vi "WireTunnel__slk_mt.vi"(8 "error in (no error)":errorcluster, 10 "vi name":string, 11 "application reference":refnum<vi>) -> (0 "error out":errorcluster)   [LabVIEW 2013, in "Lazyboots Menu Tool.lvlib"]
doc: "This VI is the core of <b>Wire Tunnel</b> function, and will be called by corresponding menu launcher."
uses:
  Library/Lazyboots Menu Tool.lvlib
  Private/WireTunnel/TypeDef_WireTunnelState__slk_mt.ctl
panel:
  # "WireTunnel__slk_mt.vi\nThis VI is the core of <b>Wire Tunnel</b> function, and will be called by corresponding menu launcher.\n\nNOTICE -- YOU MUST LEAVE THIS NOTICE IN PLACE.\n\nCopyright (c) 2011, LIANG LIU Shawn.Liu.cn@gmail.com\nAll rights reserved.\n\nRedistribution and use in source and binary forms, with or without modification, are permitted provided that the following conditions are met:\n-Redistributions of source code must retain the above copyright notice, this list of conditions and the following disclaimer.\n-Redistributions in binary form must reproduce the above copyright notice, this list of conditions and the following disclaimer in the documentation and/or other materials provided with the distribution.\n-Neither the name of the eLp nor the names of its contributors may be used to endorse or promote products derived from this software without specific prior written permission.\n\nTHIS SOFTWARE IS PROVIDED BY THE COPYRIGHT HOLDERS AND CONTRIBUTORS \"AS IS\" AND ANY EXPRESS OR IMPLIED WARRANTIES, INCLUDING, BUT NOT LIMITED TO, THE IMPLIED WARRANTIES OF MERCHANTABILITY AND FITNESS FOR A PARTICULAR PURPOSE ARE DISCLAIMED. IN NO EVENT SHALL THE COPYRIGHT HOLDER OR CONTRIBUTORS BE LIABLE FOR ANY DIRECT, INDIRECT, INCIDENTAL, SPECIAL, EXEMPLARY, OR CONSEQUENTIAL DAMAGES (INCLUDING, BUT NOT LIMITED TO, PROCUREMENT OF SUBSTITUTE GOODS OR SERVICES; LOSS OF USE, DATA, OR PROFITS; OR BUSINESS INTERRUPTION) HOWEVER CAUSED AND ON ANY THEORY OF LIABILITY, WHETHER IN CONTRACT, STRICT LIABILITY, OR TORT (INCLUDING NEGLIGENCE OR OTHERWISE) ARISING IN ANY WAY OUT OF THE USE OF THIS SOFTWARE, EVEN IF ADVISED OF THE POSSIBILITY OF SUCH DAMAGE."
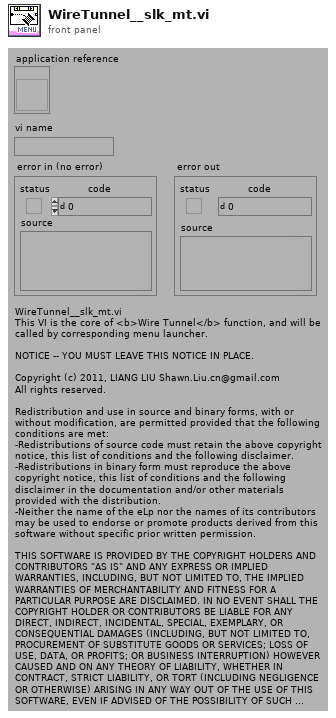
[diagram p1: front panel]
types:
  T1 = typedef "Lazyboots Menu Tool.lvlib/TypeDef_WireTunnelState__slk_mt.ctl" = enum16{"Get Menu Launch VI", "Get Tunnel Ref Array", "Wrong Selection?", "Wrong Selection", "Identify Left or Right Tunnel", "Undo.Start", "Wire Case Tunnel", "Undo.Fail/End", "End"}
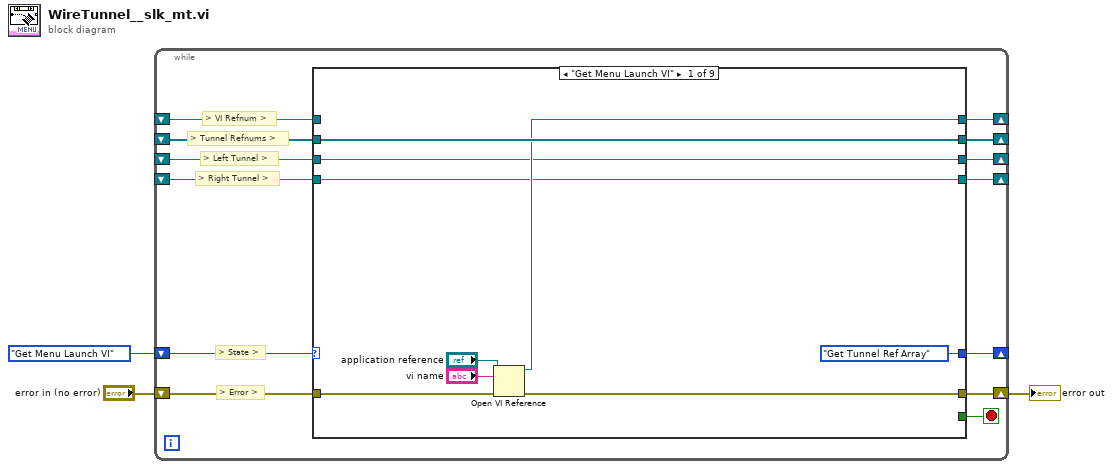
[diagram p0: block diagram]
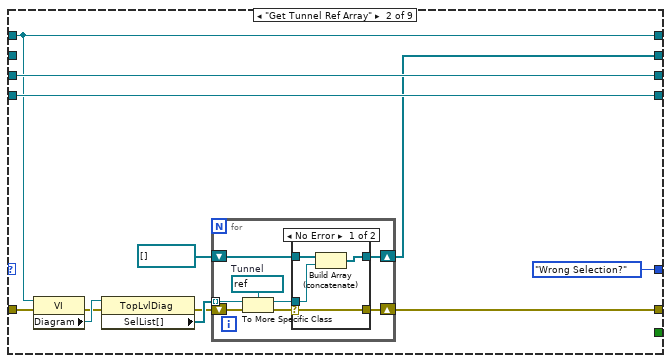
[diagram p2: hidden frame]
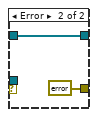
[diagram p3: hidden frame]
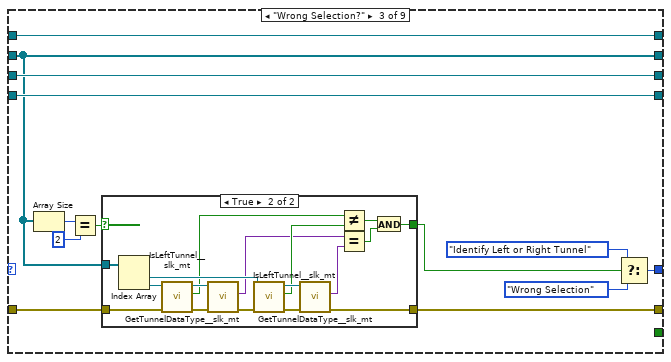
[diagram p4: hidden frame]
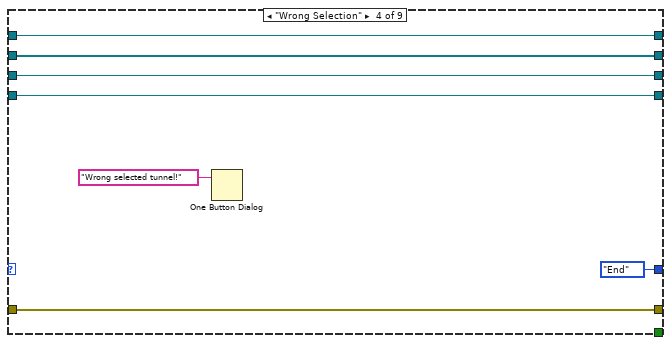
[diagram p6: hidden frame]
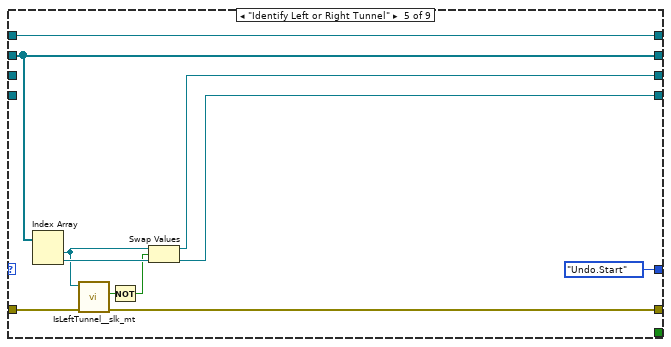
[diagram p7: hidden frame]
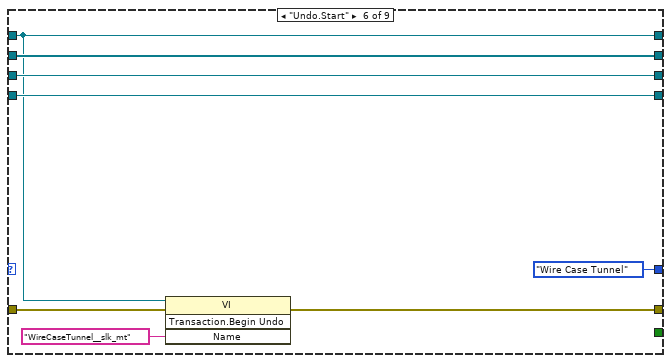
[diagram p8: hidden frame]
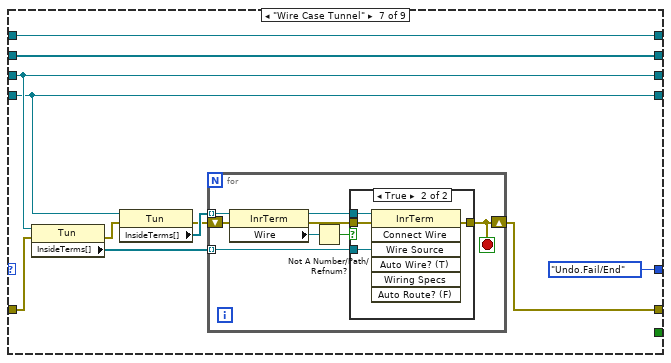
[diagram p9: hidden frame]
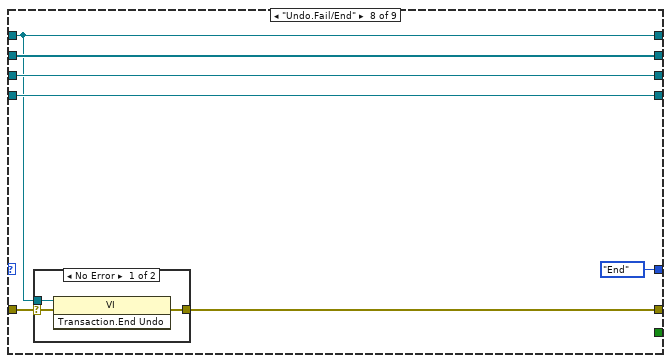
[diagram p11: hidden frame]
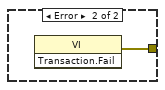
[diagram p12: hidden frame]
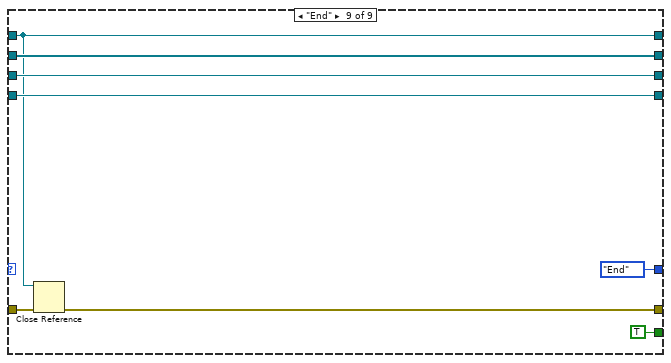
[diagram p13: hidden frame]
diagram:
  n1 = while {
    shift-right: [w13] -> _
    shift-left: TypeDef_WireTunnelState__slk_mt."Get Menu Launch VI" ("State") -> [w16]
    shift-right: [w14] -> w1
    shift-left: "error in (no error)" -> [w15]
    shift-right: [w11] -> _
    shift-left: _ -> [w12]
    shift-right: [w10] -> _
    shift-left: _ -> [w9]
    shift-right: [w7] -> _
    shift-left: _ -> [w8]
    shift-right: [w5] -> _
    shift-left: _ -> [w6]
    stop <- w4 stop-if-true
    # "> Right Tunnel >"
    # "> Left Tunnel >"
    # "> Tunnel Refnums >"
    # "> VI Refnum >"
    # "> Error >"
    # "> State >"
    n2 = case shown="\"Get Menu Launch VI\"" w16 {
      tunnel: w15 -> [w25 w29 w55 w86 w98 w105 w114 w137 w146]
      tunnel: [w22 w28 w54 w86 w97 w104 w111 w136 w147] -> w14
      tunnel: [TypeDef_WireTunnelState__slk_mt."Get Tunnel Ref Array" ("State") TypeDef_WireTunnelState__slk_mt."Wrong Selection?" ("State") w59 TypeDef_WireTunnelState__slk_mt."End" ("State") TypeDef_WireTunnelState__slk_mt."Undo.Start" ("State") TypeDef_WireTunnelState__slk_mt."Wire Case Tunnel" ("State") TypeDef_WireTunnelState__slk_mt."Undo.Fail/End" ("State") TypeDef_WireTunnelState__slk_mt."End" ("State") TypeDef_WireTunnelState__slk_mt."End" ("State")] -> w13
      tunnel: w12 -> [_ w26 w62 w88 w101 w103 w119 w135 w145]
      tunnel: [w21 w26 w62 w88 w101 w103 w119 w135 w145] -> w11
      tunnel: [w24 w27 w52 w84 w91 w109 w120 w140 w152] -> w10
      tunnel: w9 -> [w24 _ w52 w84 w91 w109 w120 w140 w152]
      tunnel: w8 -> [w20 w37 w64 w90 _ w108 w113 w139 w149]
      tunnel: [w20 w37 w64 w90 w93 w108 w113 w139 w149] -> w7
      tunnel: w6 -> [w19 w36 w63 w89 _ w107 w112 w138 w151]
      tunnel: [w19 w36 w63 w89 w92 w107 w112 w138 w151] -> w5
      tunnel: [_ _ _ _ _ _ _ _ TRUE] -> w4
      frame "Get Menu Launch VI" {
        n3 = Open VI Reference(application reference (local)="application reference", vi path="vi name", error in (no error)=w25) -> (vi reference=w21:refnum<vi>, error out=w22:errorcluster)  [unwired: 3 out]
      }
      frame "Get Tunnel Ref Array" {
        n4 = property class="VI"(reference=w26, error in=w29) -> (error out=w30:errorcluster, "Diagram"=w31:refnum<vi>)  [unwired: 1 out]
        n5 = property class="TopLvlDiag"(reference=w31, error in=w30) -> (error out=w32:errorcluster, "SelList[]"=w33:refnum<vi>[])  [unwired: 1 out]
        n6 = for {
          tunnel: w33 -> [w43] mode=indexing
          shift-right: [w38] -> w27
          shift-left: refnum<vi>[] [] -> [w39]
          shift-right: [w40] -> w28
          shift-left: w32 -> [w45]
          w44 = refnum<vi> refnum  # Tunnel
          n7 = To More Specific Class(target class=w44, reference=w43, error in=w45) -> (specific class reference=w41:refnum<vi>, error out=w42:errorcluster)
          n8 = case shown="No Error" w42 {
            selector: w42 -> [w49 _]
            tunnel: w41 -> [w46 _]
            tunnel: [w49 errorcluster {"status"=FALSE, "code"=0, "source"=""} ("error IO")] -> w40
            tunnel: w39 -> [w48 w51]
            tunnel: [w47 w51] -> w38
            frame No Error {
              n9 = Build Array (concatenate)(w48, w46) -> (w47:refnum<vi>[])
            }
            frame Error {
            }
          }
        }
      }
      frame "Wrong Selection?" {
        n10 = Array Size(array=w52) -> (size(s)=w57:i32)
        n11 = Equal?(x=w57, y=2) -> (x = y?=w58:bool)
        n12 = case shown="True" w58 {
          selector: w58 -> [w66 _]
          tunnel: w52 -> [_ w83]
          tunnel: [w65 w71] -> w54
          tunnel: [w66 w68] -> w53
          tunnel: w55 -> [w65 w67]
          frame False {
          }
          frame True {
            n13 = Index Array(array=w83) -> (element #1=w81:refnum<vi>, element #2=w82:refnum<vi>)  [unwired: 2 in]
            n14 = call "IsLeftTunnel__slk_mt.vi"("error in (no error)"=w67, "tunnel refnum in"=w82) -> ("error out"=w77:errorcluster, "left tunnel?"=w75:bool, "duplicated tunnel refnum out"=w76:refnum<vi>)  [unwired: 7 in]
            n15 = call "GetTunnelDataType__slk_mt.vi"("error in (no error)"=w77, "tunnel refnum in"=w76) -> ("error out"=w78:errorcluster, "data type"=w72:variant)  [unwired: 7 in, 1 out]
            n16 = call "IsLeftTunnel__slk_mt.vi"("error in (no error)"=w78, "tunnel refnum in"=w81) -> ("error out"=w79:errorcluster, "left tunnel?"=w74:bool, "duplicated tunnel refnum out"=w80:refnum<vi>)  [unwired: 7 in]
            n17 = call "GetTunnelDataType__slk_mt.vi"("error in (no error)"=w79, "tunnel refnum in"=w80) -> ("error out"=w71:errorcluster, "data type"=w73:variant)  [unwired: 7 in, 1 out]
            n18 = Not Equal?(x=w75, y=w74) -> (x != y?=w70:bool)
            n19 = Equal?(x=w72, y=w73) -> (x = y?=w69:bool)
            n20 = And(x=w70, y=w69) -> (x .and. y?=w68:bool)
          }
        }
        n21 = Select(t=TypeDef_WireTunnelState__slk_mt."Identify Left or Right Tunnel", s=w53, f=TypeDef_WireTunnelState__slk_mt."Wrong Selection") -> (s? t:f=w59:T1)
      }
      frame "Wrong Selection" {
        n22 = One Button Dialog(message="Wrong selected tunnel!") -> ()  [unwired: 1 in, 1 out]
      }
      frame "Identify Left or Right Tunnel" {
        n23 = Index Array(array=w91) -> (element #1=w94:refnum<vi>, element #2=w99:refnum<vi>)  [unwired: 2 in]
        n24 = call "IsLeftTunnel__slk_mt.vi"("error in (no error)"=w98, "tunnel refnum in"=w94) -> ("error out"=w97:errorcluster, "left tunnel?"=w96:bool)  [unwired: 7 in, 1 out]
        n25 = Not(x=w96) -> (.not. x?=w95:bool)
        n26 = Swap Values(12:w94, 13:w95, 14:w99) -> (1:w93:refnum<vi>, 3:w92:refnum<vi>)
      }
      frame "Undo.Start" {
        n27 = invoke class="VI" method="Transaction.Begin Undo"(reference=w103, error in=w105, "Name"="WireCaseTunnel__slk_mt") -> (error out=w104:errorcluster)  [unwired: 1 in, 3 out]
      }
      frame "Wire Case Tunnel" {
        n28 = property class="Tun"(reference=w113, error in=w114) -> (error out=w117:errorcluster, "InsideTerms[]"=w118:refnum<vi>[])  [unwired: 1 out]
        n29 = property class="Tun"(reference=w112, error in=w117) -> (error out=w115:errorcluster, "InsideTerms[]"=w116:refnum<vi>[])  [unwired: 1 out]
        n30 = for {
          shift-right: [w121] -> w111
          shift-left: w115 -> [w125]
          tunnel: w116 -> [w127] mode=indexing
          tunnel: w118 -> [w128] mode=indexing
          stop <- w121 stop-if-true
          n31 = property class="InrTerm"(reference=w127, error in=w125) -> (reference out=w126:refnum<vi>, error out=w124:errorcluster, "Wire"=w123:refnum<vi>)
          n32 = Not A Number/Path/Refnum?(number/path/refnum=w123) -> (NaN/Path/Refnum?=w122:bool)
          n33 = case shown="True" w122 {
            tunnel: w128 -> [_ w133]
            tunnel: [w129 w132] -> w121
            tunnel: w126 -> [_ w131]
            tunnel: w124 -> [w129 w130]
            frame False {
            }
            frame True {
              n34 = invoke class="InrTerm" method="Connect Wire"(reference=w131, error in=w130, "Wire Source"=w133) -> (error out=w132:errorcluster)  [unwired: 4 in, 6 out]
            }
          }
        }
      }
      frame "Undo.Fail/End" {
        n35 = case shown="No Error" w137 {
          selector: w137 -> [w143 _]
          tunnel: [w142 w144] -> w136
          tunnel: w135 -> [w141 _]
          frame No Error {
            n36 = invoke class="VI" method="Transaction.End Undo"(reference=w141, error in=w143) -> (error out=w142:errorcluster)  [unwired: 1 in, 2 out]
          }
          frame Error {
            n37 = invoke class="VI" method="Transaction.Fail"() -> (error out=w144:errorcluster)  [unwired: 3 in, 2 out]
          }
        }
      }
      frame "End" {
        n38 = Close Reference(reference=w145, error in (no error)=w146) -> (error out=w147:errorcluster)
      }
    }
  }
  "error out" <- w1
